vi "Read Flow.vi"(8 "error in (no error)":errorcluster, 11 "Bronkhorst Settings in":T1={"VISA resource name"="", "Simulated?"=FALSE, "Smoothing Steps"=1} {"Smoothing Steps" min=1 step=1}) -> (0 "error out":errorcluster, 1 "Connection Error":bool, 2 "flow":dbl, 3 "Bronkhorst Settings out":T1={"VISA resource name"="", "Simulated?"=FALSE, "Smoothing Steps"=1} {"Smoothing Steps" min=1 step=1})   [LabVIEW 2021]
uses:
  Bronkhorst M13 Flow Meter/Settings Cluster.ctl
  <vilib>/regexp/Match Regular Expression.xnode
  <vilib>/ptbypt/NI_PtbyPt.lvlib
  Bronkhorst M13 Flow Meter/Bronkhorst M13 Flow Meter.lvlib
panel:
  out "Waveform Chart":u32(graph)
  out "whole match":string
  out "x/y":dbl
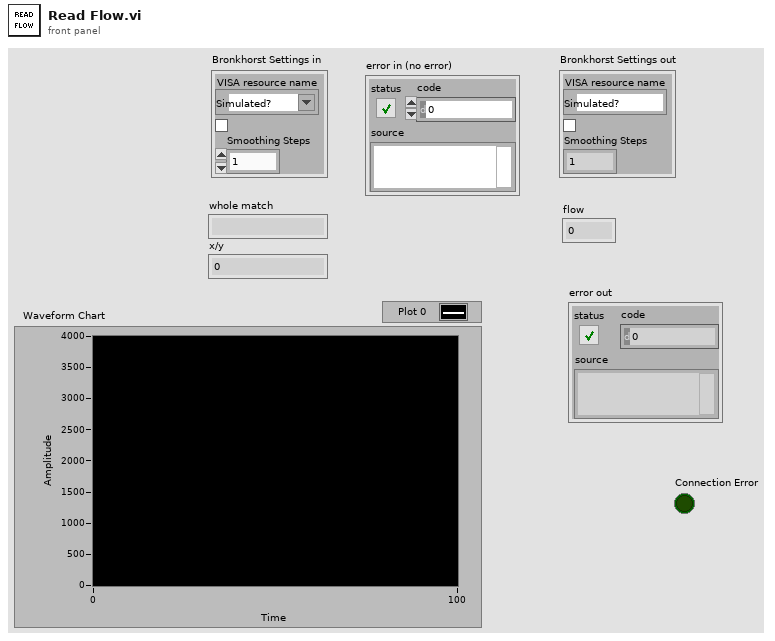
[diagram p1: front panel]
types:
  T1 = typedef "Bronkhorst M13 Flow Meter.lvlib/Settings Cluster.ctl" = cluster{"VISA resource name":refnum<visa-resource-name>, "Simulated?":bool, "Smoothing Steps":i32}
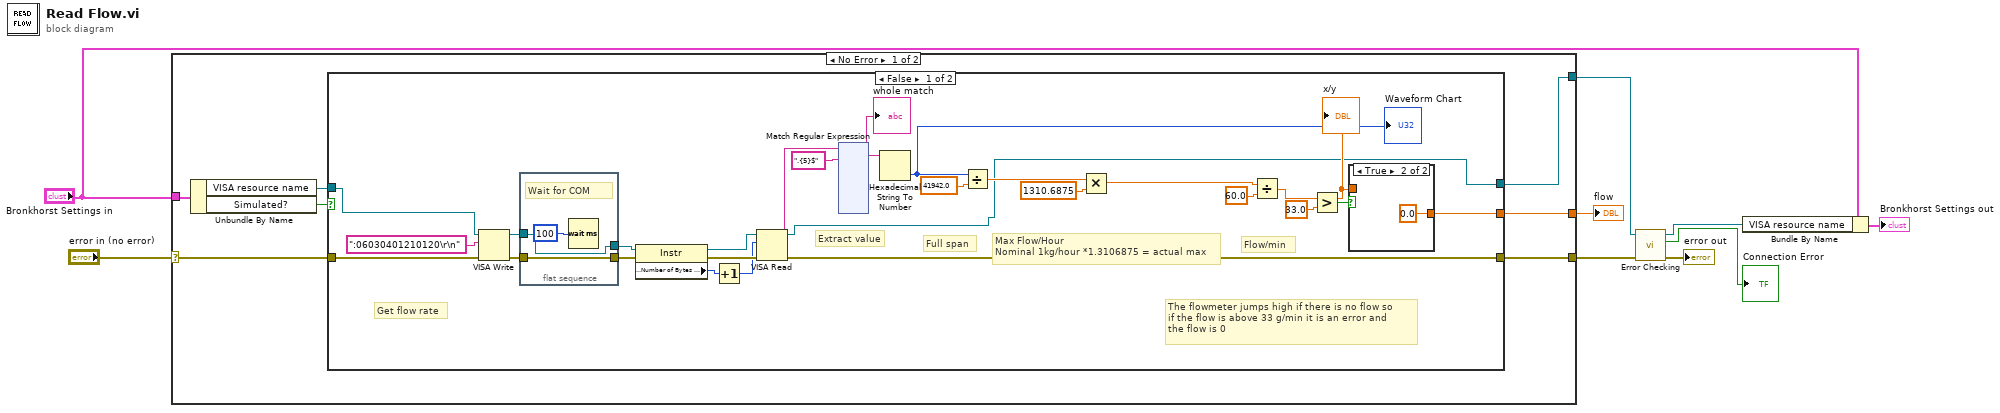
[diagram p0: block diagram]
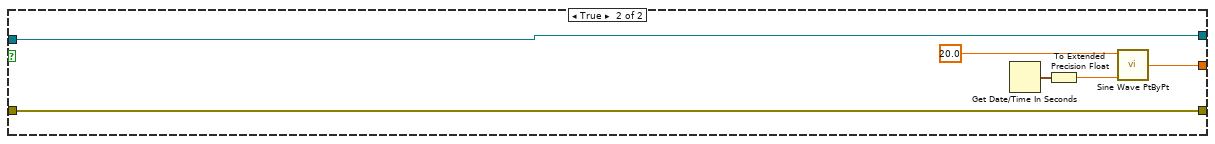
[diagram p3: hidden frame]
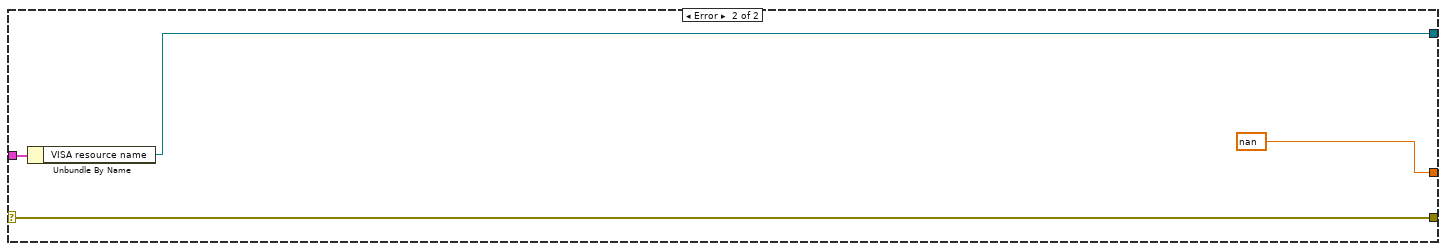
[diagram p4: hidden frame]
diagram:
  n1 = case shown="No Error" "error in (no error)" {
    selector: "error in (no error)" -> [w15 w179]
    tunnel: [w14 w179] -> w3
    tunnel: "Bronkhorst Settings in" -> [w12 w177]
    tunnel: [w13 nan ("sine wave")] -> w9
    tunnel: [w10 w176] -> w5
    frame No Error {
      n2 = Unbundle By Name(w12) -> ("VISA resource name"=w11:refnum<visa-resource-name>, "Simulated?"=w16:bool)
      n3 = case shown="False" w16 {
        tunnel: [w18 w175] -> w14
        tunnel: w15 -> [w23 w175]
        tunnel: [w27 w171] -> w13
        tunnel: [w19 w170] -> w10
        tunnel: w11 -> [w24 w170]
        frame False {
          # "Flow/min"
          # "Max Flow/Hour\nNominal 1kg/hour *1.3106875 = actual max"
          # "Full span"
          # "Extract value"
          # "Get flow rate"
          # "The flowmeter jumps high if there is no flow so \nif the flow is above 33 g/min it is an error and \nthe flow is 0"
          n4 = VISA Write(VISA resource name=w24, write buffer=":06030401210120\r\n" ("Command"), error in (no error)=w23) -> (VISA resource name out=w39:refnum<visa-resource-name>, error out=w37:errorcluster)  [unwired: 1 out]
          n5 = flat-sequence {
            tunnel: [w169] -> w38
            tunnel: w39 -> [w169]
            tunnel: [w168] -> w36
            tunnel: w37 -> [w168]
            frame #0 {
              # "Wait for COM"
              n6 = Wait (ms)(milliseconds to wait=u32 100) -> ()  [unwired: 1 out]
            }
          }
          n7 = property class="Instr"(reference=w38, error in=w36) -> (reference out=w41:refnum<visa-resource-name>, error out=w40:errorcluster, "Serial Settings:Number of Bytes at Serial Port"=w21:u32)
          n8 = Increment(x=w21) -> (x+1=w20:u32)
          n9 = VISA Read(VISA resource name=w41, byte count=w20, error in (no error)=w40) -> (VISA resource name out=w19:refnum<visa-resource-name>, read buffer=w22:string, error out=w18:errorcluster)  [unwired: 1 out]
          n10 = xnode "Match Regular Expression"("input string"=w22, "regular expression"=".{5}$" ("Regular Expression for Extracting Weight")) -> ("whole match"=w26:string)  [unwired: 4 in, 8 out]
          "whole match" <- w26
          n11 = Hexadecimal String To Number(string=w26) -> (number=w25:u32)  [unwired: 2 in, 1 out]
          "Waveform Chart" <- w25
          n12 = Divide(x=w25, y=41942.0) -> (x/y=w30:dbl)
          n13 = Multiply(x=w30, y=1310.6875) -> (x*y=w17:dbl)
          n14 = Divide(x=w17, y=60.0) -> (x/y=w28:dbl)
          "x/y" <- w28
          n15 = Greater?(x=w28, y=33.0) -> (0:w29:bool)
          n16 = case shown="True" w29 {
            tunnel: [w43 0.0] -> w27
            tunnel: w28 -> [w43 _]
            frame False {
            }
            frame True {
            }
          }
        }
        frame True {
          n17 = Get Date/Time In Seconds() -> (seconds since 1Jan1904=w174:timestamp)
          n18 = To Extended Precision Float(1:w174) -> (0:w173:ext)
          n19 = call <vilib>:"Sine Wave PtByPt.vi"("time"=w173, "amplitude"=20.0) -> ("sine wave"=w171:dbl)  [unwired: 2 in]
        }
      }
    }
    frame Error {
      n20 = Unbundle By Name(w177) -> ("VISA resource name"=w176:refnum<visa-resource-name>)
    }
  }
  "flow" <- w9
  n21 = call "Error Checking.vi"("error in (no error)"=w3, "VISA resource name"=w5) -> ("error out"=→"error out":errorcluster, "Connection Error"=→"Connection Error":bool, "VISA resource name"=w4:refnum<visa-resource-name>)  [unwired: 7 in]
  n22 = Bundle By Name(cluster="Bronkhorst Settings in", "VISA resource name"=w4) -> (→"Bronkhorst Settings out":T1)
